vi "is abstract node.vi"(8 "error in":errorcluster, 11 "TEST EDITOR in":refnum<class "TEST EDITOR.lvclass">) -> (0 "error out":errorcluster, 2 "abstract":bool, 3 "TEST EDITOR out":refnum<class "TEST EDITOR.lvclass">)   [LabVIEW 2013, in "configuration tests.lvlib" / "TEST EDITOR.lvclass"]
uses:
  TEST EDITOR.lvclass
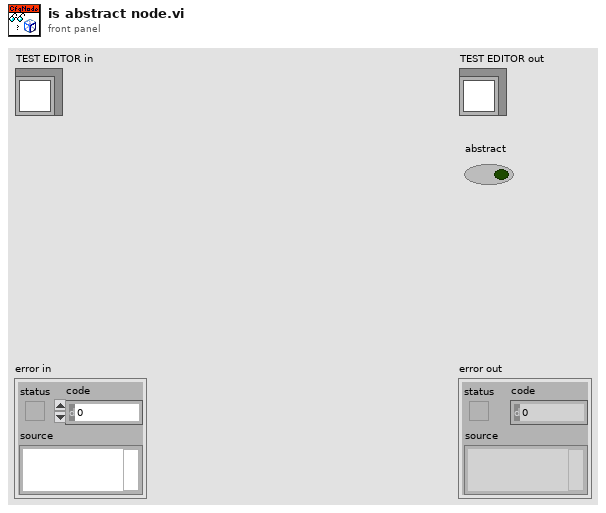
[diagram p1: front panel]
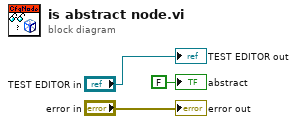
[diagram p0: block diagram]
diagram:
  "error out" <- "error in"
  "TEST EDITOR out" <- "TEST EDITOR in"
  "abstract" <- FALSE ("abstract")
